vi "Read Sample Push State.vi"(8 "error in (no error)":errorcluster, 9 "State Timeout (Inf)":dbl=inf, 10 "Reinit Timer (F)":bool caption="Reset", 11 "cRIO-CO2 in":refnum<class "cRIO-CO2.lvclass">) -> (0 "error out":errorcluster, 1 "Sample Push State":string, 2 "Sample Push State":T2=enum."Idle", 3 "cRIO-CO2 out":refnum<class "cRIO-CO2.lvclass">, 4 "Timeout?":bool, 5 "Source Storage":T1, 6 "Elapsed Time (s)":dbl)   [LabVIEW 2015, in "cRIO-Carbondioxide.lvlib" / "cRIO-CO2.lvlib" / "cRIO-CO2.lvclass"]
uses:
  cRIO-CO2.lvclass
  Controls/Sample Push State Enumerator.ctl
  Controls/Sample Transfer Container Enumerator.ctl
  cRIO-CO2.lvclass/cRIO-CO2.ctl
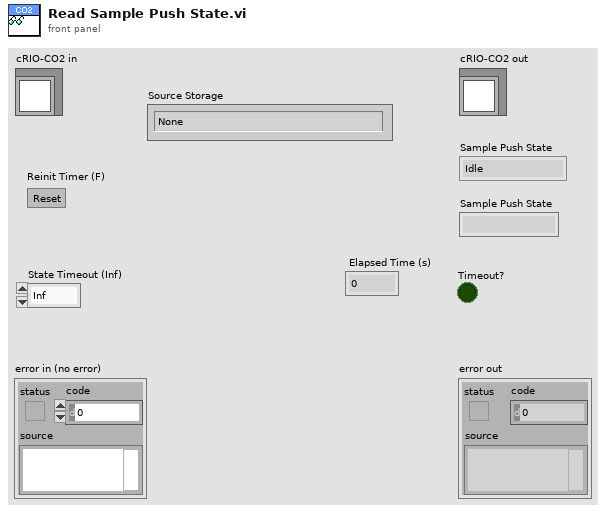
[diagram p1: front panel]
types:
  T1 = typedef "Sample Transfer Container Enumerator.ctl" = enum16{"None", "Sample 1", "Sample 2", "Sample 3", "Sample 4", "Sample 5", "Storage 01", "Storage 02", "Storage 03", "Storage 04", "Storage 05", "Storage 06", "Storage 07", "Storage 08", "Storage 09", "Storage 10", "Storage 11", "Storage 12", "Syringe", "Undefined"}
  T2 = typedef "Sample Push State Enumerator.ctl" = enum16{"Undefined", "Initialize", "Dilute", "Close Transfer Line", "Start Heaters", "Warm Up Syringe", "Ready to Push", "Push", "Initiate Stash", "Stash", "Complete", "Abort", "Idle", "Error"}
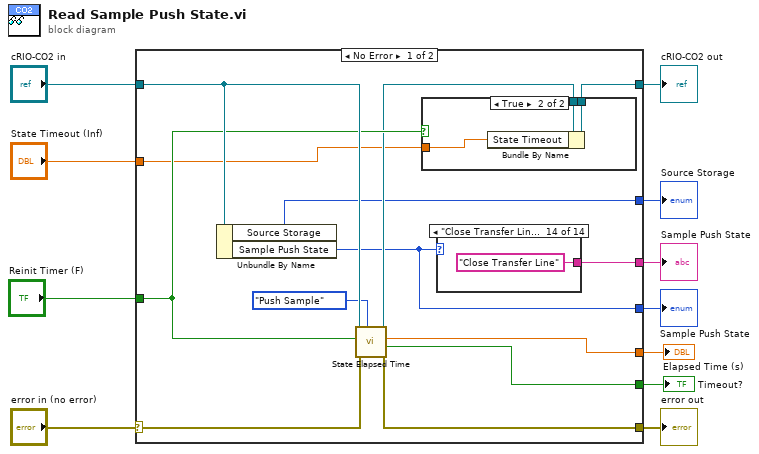
[diagram p0: block diagram]
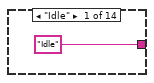
[diagram p3: hidden frame]
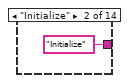
[diagram p4: hidden frame]
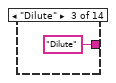
[diagram p5: hidden frame]
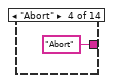
[diagram p6: hidden frame]
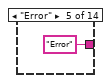
[diagram p7: hidden frame]
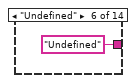
[diagram p8: hidden frame]
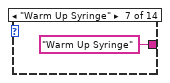
[diagram p9: hidden frame]
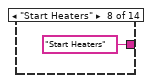
[diagram p10: hidden frame]
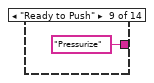
[diagram p11: hidden frame]
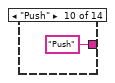
[diagram p12: hidden frame]
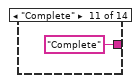
[diagram p13: hidden frame]
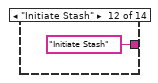
[diagram p14: hidden frame]
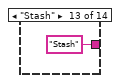
[diagram p15: hidden frame]
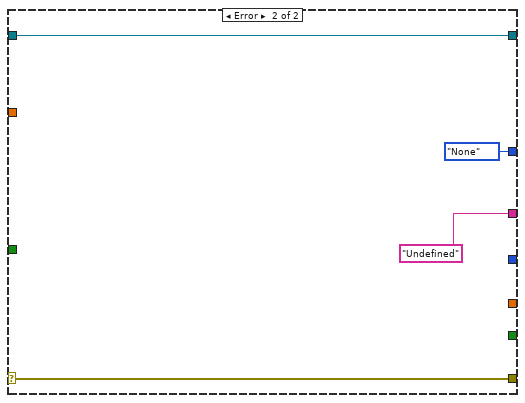
[diagram p16: hidden frame]
diagram:
  n1 = case shown="No Error" "error in (no error)" {
    selector: "error in (no error)" -> [w21 w45]
    tunnel: [w20 w45] -> w10
    tunnel: [w17 w46] -> w8
    tunnel: "cRIO-CO2 in" -> [w22 w46]
    tunnel: [w14 _] -> w7
    tunnel: [w24 "Undefined"] -> w6
    tunnel: [w23 _] -> w5
    tunnel: "Reinit Timer (F)" -> [w19 _]
    tunnel: "State Timeout (Inf)" -> [w16 _]
    tunnel: [w13 _] -> w2
    tunnel: [w12 Sample_Transfer_Container_Enumerator."None" ("Source Storage")] -> w1
    frame No Error {
      n2 = Unbundle By Name(w22) -> ("Source Storage"=w12:T1, "Sample Push State"=w14:T2)
      n3 = call "State Elapsed Time.vi"("State Machine"=enum16{"Transfer Sample", "Push Sample"}."Push Sample", "error in (no error)"=w21, "Reset (F)"=w19, "cRIO-CO2 in"=w22) -> ("error out"=w20:errorcluster, "State Timeout?"=w23:bool, "Elapsed Time (s)"=w13:dbl, "cRIO-CO2 out"=w18:refnum<class "cRIO-CO2.lvclass">)  [unwired: 4 in]
      n4 = case shown="True" w19 {
        tunnel: w18 -> [w25 w28]
        tunnel: [w25 w27] -> w17
        tunnel: w16 -> [_ w26]
        frame False {
        }
        frame True {
          n5 = Bundle By Name(cluster=w28, "State Timeout"=w26) -> (w27:refnum<class "cRIO-CO2.lvclass">)
        }
      }
      n6 = case shown="\"Close Transfer Line\"" w14 {
        tunnel: ["Idle" "Initialize" "Dilute" "Abort" "Error" "Undefined" "Warm Up Syringe" "Start Heaters" "Pressurize" "Push" "Complete" "Initiate Stash" "Stash" "Close Transfer Line"] -> w24
        frame "Idle" {
        }
        frame "Initialize" {
        }
        frame "Dilute" {
        }
        frame "Abort" {
        }
        frame "Error" {
        }
        frame "Undefined" {
        }
        frame "Warm Up Syringe" {
        }
        frame "Start Heaters" {
        }
        frame "Ready to Push" {
        }
        frame "Push" {
        }
        frame "Complete" {
        }
        frame "Initiate Stash" {
        }
        frame "Stash" {
        }
        frame "Close Transfer Line" {
        }
      }
    }
    frame Error {
    }
  }
  "error out" <- w10
  "cRIO-CO2 out" <- w8
  "Sample Push State" <- w7
  "Sample Push State" <- w6
  "Timeout?" <- w5
  "Elapsed Time (s)" <- w2
  "Source Storage" <- w1
